vi "Initialize.vi"(8 "error in (no error)":errorcluster, 11 "Controller Actor.lvlib:Controller.lvclass":refnum<class "Controller.lvclass">) -> (0 "error out":errorcluster, 2 "stop event out":refnum<user-event>, 3 "Controller out":refnum<class "Controller.lvclass">)   [LabVIEW 2026, in "Controller Actor.lvlib" / "Controller.lvclass"]
uses:
  Controller.lvclass
  C:/Program Files/National Instruments/LabVIEW 2026/vi.lib/ActorFramework/Actor/Actor.lvclass
  <vilib>/ActorFramework/Actor/Actor.lvclass/Actor.ctl
  <vilib>/ActorFramework/Message Enqueuer/Message Enqueuer.lvclass/Message Enqueuer.ctl
  Controller Messages/Update lookup table of devices on system Msg/Update lookup table of devices on system Msg.lvclass/Update lookup table of devices on system Msg.ctl
  Controller.lvclass/Controller.ctl
  <vilib>/ActorFramework/Message Enqueuer/Init from Existing Queue.vi
  <vilib>/ActorFramework/Message Enqueuer/Enqueue.vi
  Messages/Measurements Scan Msg/Measurements Scan Msg.lvclass
  C:/Program Files/National Instruments/LabVIEW 2026/vi.lib/ActorFramework/Message/Message.lvclass
  Controller Messages/Update lookup table of devices on system Msg/Update lookup table of devices on system Msg.lvclass
  <vilib>/ActorFramework/Message Priority Queue/Priority Enqueue.vi
  <vilib>/ActorFramework/Message Enqueuer/Message Enqueuer.lvclass
  <vilib>/ActorFramework/Actor/Actor.lvclass
  Messages/Scan Hardware Message/Scan Hardware Message.lvclass
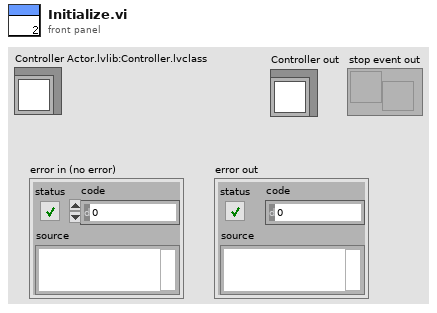
[diagram p1: front panel]
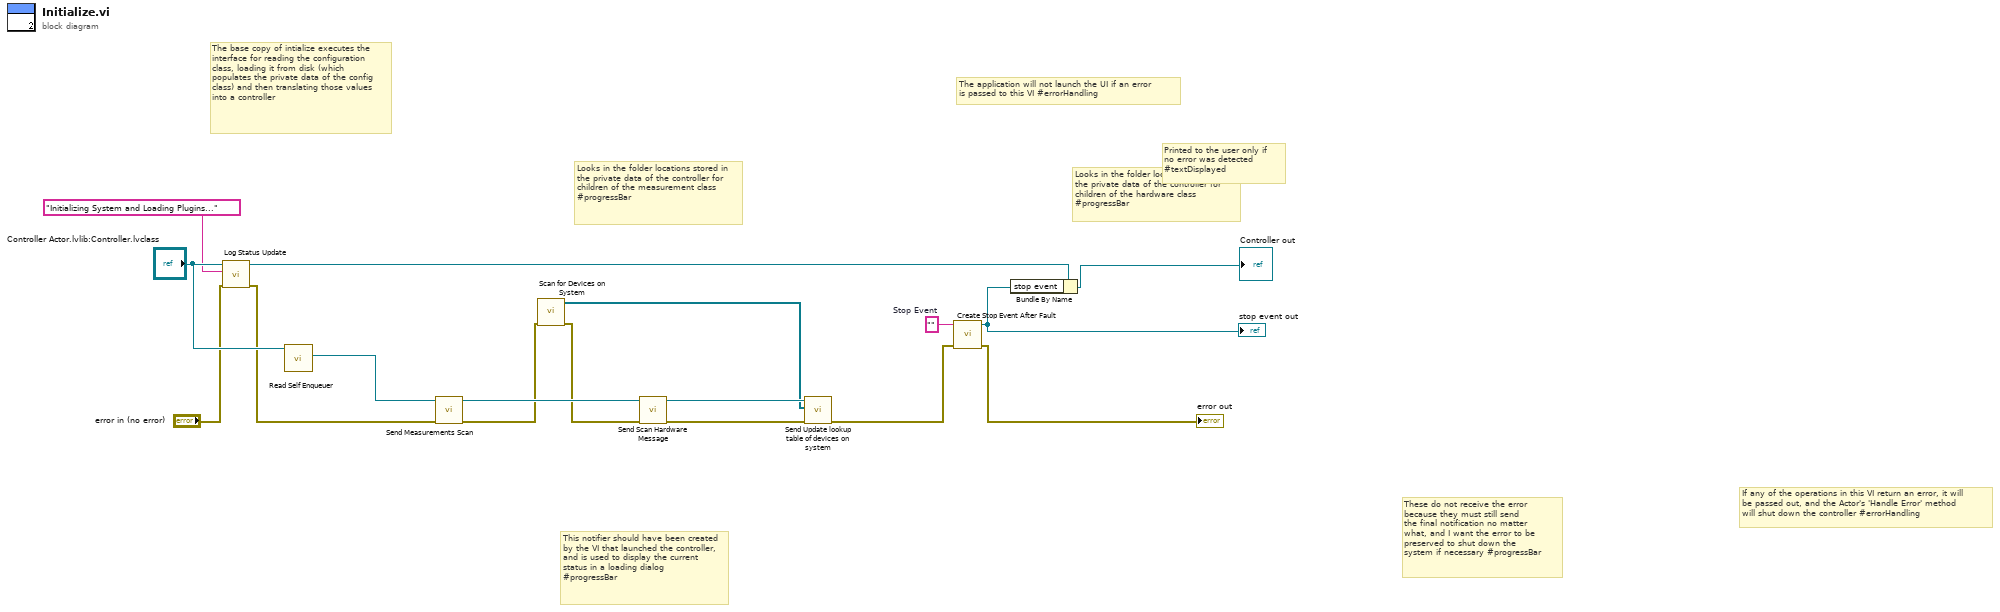
[diagram p0: block diagram]
diagram:
  w11 = ""  # Stop Event
  # "The base copy of intialize executes the interface for reading the configuration class, loading it from disk (which populates the private data of the config class) and then translating those values into a controller"
  # "Printed to the user only if \nno error was detected\n#textDisplayed"
  # "This notifier should have been created by the VI that launched the controller, and is used to display the current status in a loading dialog #progressBar"
  # "Looks in the folder locations stored in the private data of the controller for children of the hardware class \n#progressBar"
  # "Looks in the folder locations stored in the private data of the controller for children of the measurement class #progressBar"
  # "These do not receive the error\nbecause they must still send \nthe final notification no matter \nwhat, and I want the error to be \npreserved to shut down the \nsystem if necessary #progressBar"
  # "The application will not launch the UI if an error\nis passed to this VI #errorHandling"
  # "If any of the operations in this VI return an error, it will\nbe passed out, and the Actor's 'Handle Error' method \nwill shut down the controller #errorHandling"
  n1 = call-dynamic "Log Status Update.vi"("error in (no error)"="error in (no error)", "String"="Initializing System and Loading Plugins...", "Controller in"="Controller Actor.lvlib:Controller.lvclass") -> ("error out"=w12:errorcluster, "Controller out"=w10:refnum<class "Controller.lvclass">)  [unwired: 7 in]
  n2 = call <vilib>:"Read Self Enqueuer.vi"("Actor"="Controller Actor.lvlib:Controller.lvclass") -> ("Self Enqueuer"=w13:refnum<class "Message Enqueuer.lvclass">)  [unwired: 10 in]
  n3 = call "Send Measurements Scan.vi"("error in (no error)"=w12, "Message Enqueuer"=w13) -> ("error out"=w6:errorcluster, "Message Enqueuer out"=w17:refnum<class "Message Enqueuer.lvclass">)  [unwired: 8 in]
  n4 = call "Scan for Devices on System.vi"("error in (no error)"=w6) -> ("error out"=w5:errorcluster, "Resources out"=w3:refnum<k20>[])  [unwired: 8 in, 1 out]
  n5 = call "Send Scan Hardware Message.vi"("error in (no error)"=w5, "Message Enqueuer in"=w17) -> ("error out"=w2:errorcluster, "Message Enqueuer out"=w4:refnum<class "Message Enqueuer.lvclass">)  [unwired: 8 in]
  n6 = call "Send Update lookup table of devices on system.vi"("error in (no error)"=w2, "Hardware Resources"=w3, "Message Enqueuer"=w4) -> ("error out"=w1:errorcluster)  [unwired: 7 in, 1 out]
  n7 = call "Create Stop Event After Fault.vi"("error in"=w1, "user event datatype"=w11) -> ("error out"=→"error out":errorcluster, "user event"=w9:refnum<user-event>)  [unwired: 8 in]
  "stop event out" <- w9
  n8 = Bundle By Name(cluster=w10, "stop event"=w9) -> (→"Controller out":refnum<class "Controller.lvclass">)
